vi "Remote Shutdown.vi"(8 "error out":errorcluster, 10 "Init?":bool, 11 "port":refnum<k16>) -> (0 "error out 2":errorcluster, 1 "REMOTE STOP":T1, 2 "Shutdown?":bool, 3 "port 2":refnum<k16>)   [LabVIEW 2015]
uses:
  Remote Stop Type.ctl
  Global Data.vi
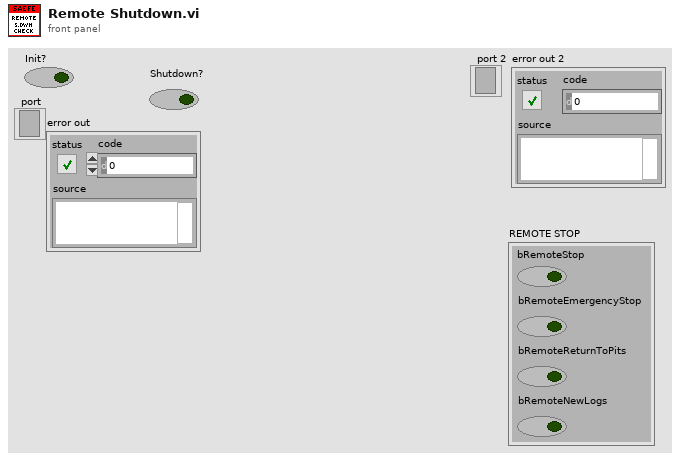
[diagram p1: front panel]
types:
  T1 = typedef "Remote Stop Type.ctl" = cluster{"bRemoteStop":bool, "bRemoteEmergencyStop":bool, "bRemoteReturnToPits":bool, "bRemoteNewLogs":bool}
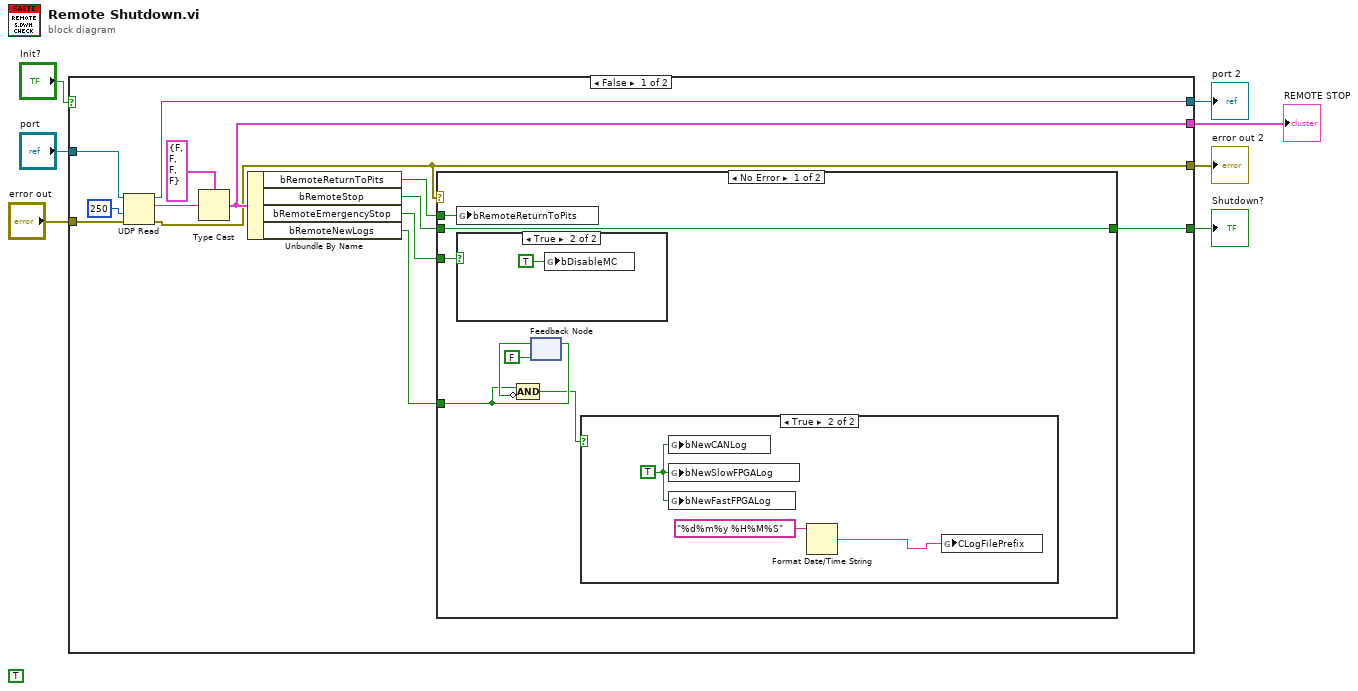
[diagram p0: block diagram]
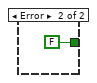
[diagram p4: hidden frame]
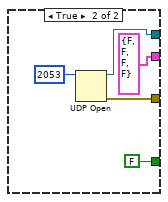
[diagram p5: hidden frame]
diagram:
  (unwired) TRUE
  n1 = case shown="False" "Init?" {
    tunnel: [w18 w36] -> w4
    tunnel: [w11 w35] -> w3
    tunnel: "port" -> [w20 _]
    tunnel: "error out" -> [w19 _]
    tunnel: [w9 FALSE] -> w2
    tunnel: [w14 T1 {"bRemoteStop"=FALSE, "bRemoteEmergencyStop"=FALSE, "bRemoteReturnToPits"=FALSE, "bRemoteNewLogs"=FALSE} ("REMOTE STOP")] -> w1
    frame False {
      n2 = UDP Read(connection ID=w20, timeout ms (25000)=250, 8:w19) -> (data out=w16:string, error out=w11:errorcluster, 3:w18:refnum<k16>)  [unwired: 1 in, 2 out]
      n3 = Type Cast(type=T1 {"bRemoteStop"=FALSE, "bRemoteEmergencyStop"=FALSE, "bRemoteReturnToPits"=FALSE, "bRemoteNewLogs"=FALSE} ("REMOTE STOP"), x=w16) -> (*(type *) &x=w14:T1)
      n4 = Unbundle By Name(w14) -> ("bRemoteReturnToPits"=w13:bool, "bRemoteStop"=w10:bool, "bRemoteEmergencyStop"=w12:bool, "bRemoteNewLogs"=w8:bool)
      n5 = case shown="No Error" w11 {
        tunnel: w13 -> [w27 _]
        tunnel: w12 -> [w26 _]
        tunnel: w10 -> [w25 _]
        tunnel: [w25 FALSE ("REMOTE STOP")] -> w9
        tunnel: w8 -> [w22 _]
        frame No Error {
          n6 = global write "Global Data.vi" "bRemoteReturnToPits"(w27) -> ()
          n7 = case shown="True" w26 {
            frame False {
            }
            frame True {
              n8 = global write "Global Data.vi" "bDisableMC"(TRUE ("Disable MC")) -> ()
            }
          }
          n9 = feedback-in #1(w22) -> ()
          n10 = feedback #1(FALSE ("New TDMS Files")) -> (w23:bool)
          n11 = Compound Arithmetic op=AND(w22, invert w23) -> (w21:bool)
          n12 = case shown="True" w21 {
            frame False {
            }
            frame True {
              w30 = TRUE ("New MC TDMS")
              n13 = global write "Global Data.vi" "bNewCANLog"(w30) -> ()
              n14 = global write "Global Data.vi" "bNewSlowFPGALog"(w30) -> ()
              n15 = global write "Global Data.vi" "bNewFastFPGALog"(w30) -> ()
              n16 = Format Date/Time String(time format string (%c)="%d%m%y %H%M%S") -> (date/time string=w28:string)  [unwired: 2 in]
              n17 = global write "Global Data.vi" "CLogFilePrefix"(w28) -> ()
            }
          }
        }
        frame Error {
        }
      }
    }
    frame True {
      n18 = UDP Open(11:u16 2053 ("port")) -> (port=w36:refnum<k16>, 0:w35:errorcluster)  [unwired: 4 in, 1 out]
    }
  }
  "Shutdown?" <- w2
  "port 2" <- w4
  "error out 2" <- w3
  "REMOTE STOP" <- w1
